vi "PCB Coverage graph.vi"(0 "UpdatedData":T1, 5 "error in (no error)":errorcluster, 6 "XY Graph":refnum<vi>, 7 "index":i32, 9 "Disable Autoscale":bool, 13 "Initialise graph":bool=TRUE) -> (19 "error out":errorcluster)   [LabVIEW 2018, in "Manipulate IPF.lvlib"]
uses:
  Manipulate IPF.lvlib
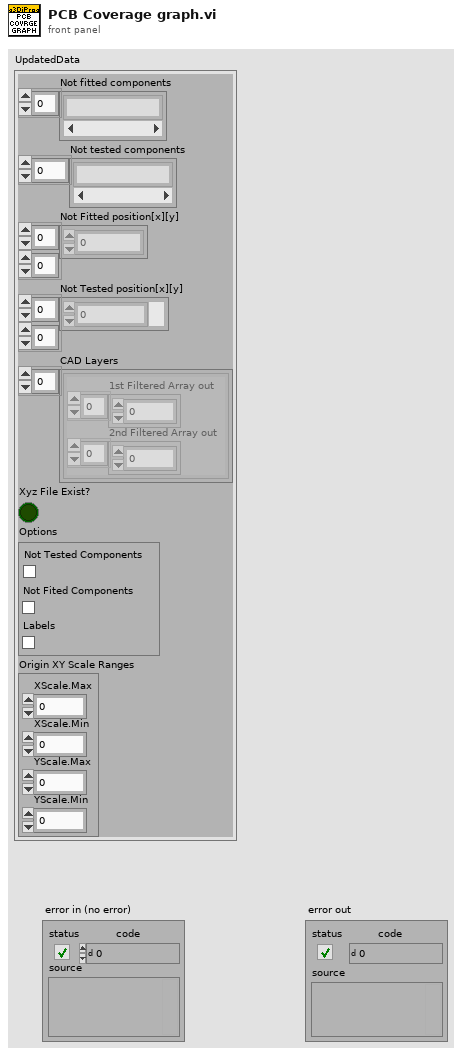
[diagram p1: front panel]
types:
  T1 = cluster{"Not fitted components":string[], "Not tested components":string[], "Not Fitted position[x][y] ":dbl[][], "Not Tested position[x][y]":dbl[][], "CAD Layers":cluster{"1st Filtered Array out":sgl[], "2nd Filtered Array out":sgl[]}[], "Xyz File Exist? ":bool, "Options":cluster{"Enable Not Tested Components":bool, "Enable Not Fited Components":bool, "Enable Labels":bool}, "Origin XY Scale Ranges":cluster{"XScale.Max":dbl, "XScale.Min":dbl, "YScale.Max":dbl, "YScale.Min":dbl}}
  T2 = cluster{"1st Filtered Array out":sgl[], "2nd Filtered Array out":sgl[]}[]
  T3 = cluster{"1st Filtered Array out":sgl[], "2nd Filtered Array out":sgl[]}
  T4 = cluster{"X Array Out":dbl[], "Y Array out":dbl[]}
  T5 = cluster{"X Array Out":dbl[], "Y Array out":dbl[]}[]
  T6 = typedef "LVPoint32TypeDef.ctl" = cluster{"Horizontal":i32, "Vertical":i32}
  T7 = typedef "LVAnnotationListTypeDef.ctl" = cluster{"Name":string, "Color":u32, "Style":u8, "Point Style":u8, "Name Visible":bool, "Allow Drag":bool, "Annotation Mode":u32, "Plot":i32, "Index":i32, "Position":cluster{"X":dbl, "Y":dbl}, "X Scale":u32, "Y Scale":u32, "Show Arrow":bool, "Lock Name":bool, "Plot Area":i32, "Label Offset":cluster{"X":dbl, "Y":dbl}}[]
  T8 = cluster{"Name":string, "Color":u32, "Style":u8, "Point Style":u8, "Name Visible":bool, "Allow Drag":bool, "Annotation Mode":u32, "Plot":i32, "Index":i32, "Position":cluster{"X":dbl, "Y":dbl}, "X Scale":u32, "Y Scale":u32, "Show Arrow":bool, "Lock Name":bool, "Plot Area":i32, "Label Offset":cluster{"X":dbl, "Y":dbl}}
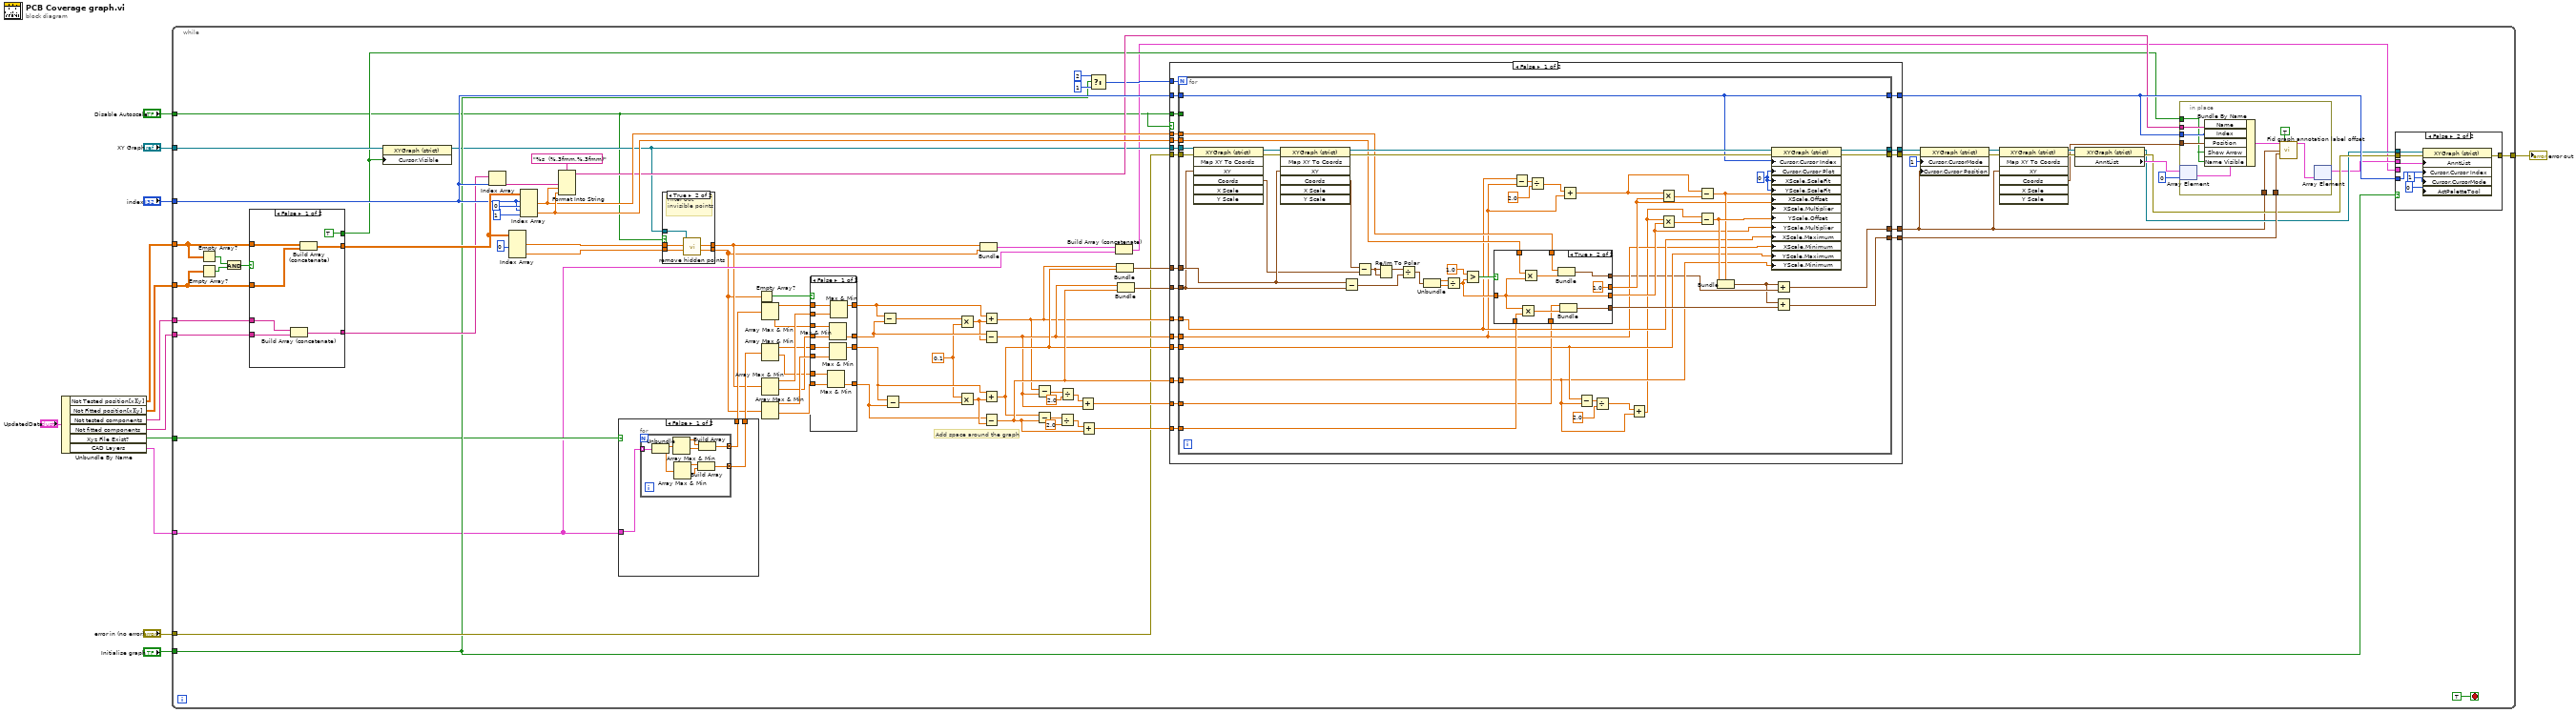
[diagram p0: block diagram]
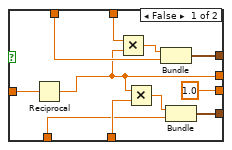
[diagram p2: hidden frame]
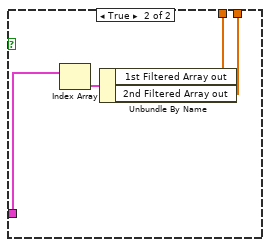
[diagram p4: hidden frame]
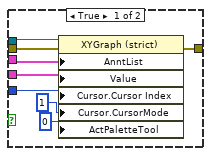
[diagram p7: hidden frame]
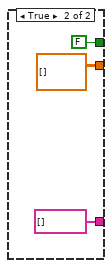
[diagram p8: hidden frame]
diagram:
  n1 = Unbundle By Name("UpdatedData") -> ("Not Tested position[x][y]"=w4:dbl[][], "Not Fitted position[x][y]"=w2:dbl[][], "Not tested components"=w3:string[], "Not fitted components"=w1:string[], "Xyz File Exist?"=w6:bool, "CAD Layers"=w7:T2)
  n2 = while {
    tunnel: "error in (no error)" -> [w71]
    tunnel: w4 -> [w62]
    tunnel: "index" -> [w49]
    tunnel: "XY Graph" -> [w57]
    tunnel: [w64] -> w10
    tunnel: "Initialise graph" -> [w33]
    tunnel: w2 -> [w61]
    tunnel: w3 -> [w54]
    tunnel: w1 -> [w53]
    tunnel: "Disable Autoscale" -> [w14]
    tunnel: w6 -> [w20]
    tunnel: w7 -> [w19]
    stop <- TRUE stop-if-true
    w98 = 0.1
    # "Add space around the graph"
    n3 = Empty Array?(array=w62) -> (empty?=w60:bool)
    n4 = Empty Array?(array=w61) -> (empty?=w59:bool)
    n5 = And(x=w60, y=w59) -> (x .and. y?=w58:bool)
    n6 = case shown="False" w58 {
      tunnel: w62 -> [w264 _]
      tunnel: w61 -> [w263 _]
      tunnel: [w262 dbl[][] []] -> w56
      tunnel: [TRUE FALSE] -> w30
      tunnel: w54 -> [w261 _]
      tunnel: w53 -> [w260 _]
      tunnel: [w259 string[] []] -> w48
      frame False {
        n7 = Build Array (concatenate)(w261, w260) -> (w259:string[])
        n8 = Build Array (concatenate)(w264, w263) -> (w262:dbl[][])
      }
      frame True {
      }
    }
    n9 = property class="XYGraph (strict)"(reference=w57, "Cursor.Visible"=w30) -> (reference out=w24:refnum<vi>)  [unwired: 1 in, 1 out]
    n10 = Index Array(array=w48, index=w49) -> (element=w47:string)
    n11 = Index Array(array=w56, index (col) #1=0 ("index (row)")) -> (element #1=w23:dbl[], element #2=w22:dbl[])  [unwired: 3 in]
    n12 = Index Array(array=w56, index (row) #1=w49, index (col) #1=0 ("index (row)"), index (row) #2=w49, index (col) #2=1 ("index (row)")) -> (element #1=w50:dbl, element #2=w51:dbl)
    n13 = Format Into String(format string="%s  (%.3fmm,%.3fmm)", w47, w50, w51) -> (resulting string=w39:string)  [unwired: 2 in, 1 out]
    n14 = case shown="False" w20 {
      tunnel: [w196 w207] -> w27
      tunnel: [w197 w208] -> w28
      tunnel: w19 -> [w195 w210]
      frame False {
        n15 = for {
          tunnel: w195 -> [w206] mode=indexing
          tunnel: [w202] -> w197 mode=concatenating
          tunnel: [w198] -> w196 mode=concatenating
          n16 = Unbundle(w206) -> ("1st Filtered Array out"=w205:sgl[], "2nd Filtered Array out"=w201:sgl[])
          n17 = Array Max & Min(array=w205) -> (max value=w204:sgl, min value=w203:sgl)  [unwired: 2 out]
          n18 = Array Max & Min(array=w201) -> (max value=w199:sgl, min value=w200:sgl)  [unwired: 2 out]
          n19 = Build Array(w199, w200) -> (w198:sgl[])
          n20 = Build Array(w204, w203) -> (w202:sgl[])
        }
      }
      frame True {
        n21 = Index Array(array=w210) -> (element=w209:T3)  [unwired: 1 in]
        n22 = Unbundle By Name(w209) -> ("1st Filtered Array out"=w208:sgl[], "2nd Filtered Array out"=w207:sgl[])
      }
    }
    n23 = case shown="True" w14 {
      tunnel: w24 -> [_ w217]
      tunnel: w23 -> [w212 w214]
      tunnel: w22 -> [w211 w213]
      tunnel: [w211 w215] -> w15
      tunnel: [w212 w216] -> w16
      frame False {
      }
      frame True {
        # "Filter out invisible points"
        n24 = call "remove hidden points.vi"("Y Array in"=w213, "X Array In"=w214, "XYGraph in"=w217) -> ("Y Array out"=w215:dbl[], "X Array Out"=w216:dbl[])  [unwired: 6 in, 1 out]
      }
    }
    n25 = Empty Array?(array=w15) -> (empty?=w55:bool)
    n26 = Array Max & Min(array=w28) -> (max value=w86:sgl, min value=w87:sgl)  [unwired: 2 out]
    n27 = Array Max & Min(array=w27) -> (max value=w88:sgl, min value=w89:sgl)  [unwired: 2 out]
    n28 = Array Max & Min(array=w16) -> (max value=w90:dbl, min value=w91:dbl)  [unwired: 2 out]
    n29 = Array Max & Min(array=w15) -> (max value=w93:dbl, min value=w92:dbl)  [unwired: 2 out]
    n30 = case shown="False" w55 {
      tunnel: [w229 w230] -> w31
      tunnel: [w228 w231] -> w100
      tunnel: [w227 w232] -> w99
      tunnel: [w226 w233] -> w32
      tunnel: w93 -> [w225 _]
      tunnel: w92 -> [w224 _]
      tunnel: w91 -> [w223 _]
      tunnel: w90 -> [w222 _]
      tunnel: w89 -> [w221 w230]
      tunnel: w88 -> [w220 w231]
      tunnel: w87 -> [w219 w232]
      tunnel: w86 -> [w218 w233]
      frame False {
        n31 = Max & Min(x=w221, y=w224) -> (min(x,y)=w229:dbl)  [unwired: 1 out]
        n32 = Max & Min(x=w219, y=w223) -> (min(x,y)=w227:dbl)  [unwired: 1 out]
        n33 = Max & Min(x=w220, y=w225) -> (max(x,y)=w228:dbl)  [unwired: 1 out]
        n34 = Max & Min(x=w218, y=w222) -> (max(x,y)=w226:dbl)  [unwired: 1 out]
      }
      frame True {
      }
    }
    n35 = Subtract(x=w32, y=w99) -> (x-y=w94:dbl)
    n36 = Subtract(x=w100, y=w31) -> (x-y=w95:dbl)
    n37 = Multiply(x=w94, y=w98) -> (x*y=w96:dbl)
    n38 = Multiply(x=w98, y=w95) -> (x*y=w97:dbl)
    n39 = Bundle("X Array Out"=w16, "Y Array out"=w15) -> (w21:T4)  [unwired: 1 in]
    n40 = Add(x=w32, y=w96) -> (x+y=w74:dbl)
    n41 = Subtract(x=w99, y=w96) -> (x-y=w75:dbl)
    n42 = Add(x=w100, y=w97) -> (x+y=w76:dbl)
    n43 = Subtract(x=w31, y=w97) -> (x-y=w77:dbl)
    n44 = Subtract(x=w74, y=w75) -> (x-y=w80:dbl)
    n45 = Subtract(x=w76, y=w77) -> (x-y=w85:dbl)
    n46 = Divide(x=w85, y=2.0) -> (x/y=w83:dbl)
    n47 = Divide(x=w80, y=2.0) -> (x/y=w82:dbl)
    n48 = Add(x=w82, y=w75) -> (x+y=w78:dbl)
    n49 = Add(x=w83, y=w77) -> (x+y=w79:dbl)
    n50 = Select(t=2, s=w33, f=1) -> (s? t:f=w35:i32)
    n51 = Build Array (concatenate)(w21, w19) -> (w17:T5)
    n52 = Bundle(w74, w76) -> (w72:cluster{dbl, dbl})  [unwired: 1 in]
    n53 = Bundle(w75, w77) -> (w73:cluster{dbl, dbl})  [unwired: 1 in]
    n54 = case shown="False" w14 {
      tunnel: w79 -> [w120 _]
      tunnel: w78 -> [w119 _]
      tunnel: w77 -> [w118 _]
      tunnel: w76 -> [w117 _]
      tunnel: w75 -> [w116 _]
      tunnel: w74 -> [w115 _]
      tunnel: w73 -> [w114 _]
      tunnel: w72 -> [w113 _]
      tunnel: w71 -> [w112 w192]
      tunnel: [w111 w192] -> w66
      tunnel: w51 -> [w110 _]
      tunnel: w50 -> [w109 _]
      tunnel: w49 -> [w108 w194]
      tunnel: [w107 _] -> w42
      tunnel: [w106 w194] -> w41
      tunnel: w35 -> [w105 _]
      tunnel: [w104 w193] -> w26
      tunnel: [w103 _] -> w25
      tunnel: w24 -> [w102 w193]
      tunnel: w14 -> [w101 _]
      frame False {
        n55 = for {
          N: w105 -> [_]
          tunnel: w113 -> [w170]
          tunnel: w114 -> [w169]
          tunnel: w120 -> [w168]
          tunnel: w109 -> [w147]
          tunnel: w110 -> [w148]
          tunnel: w119 -> [w130]
          tunnel: w112 -> [w167]
          tunnel: w102 -> [w166]
          tunnel: [w123] -> w103
          tunnel: [w122] -> w107
          tunnel: [w151] -> w104
          tunnel: [w126] -> w111
          tunnel: w115 -> [w138]
          tunnel: w116 -> [w136]
          tunnel: w117 -> [w129]
          tunnel: w118 -> [w128]
          tunnel: w108 -> [w149]
          tunnel: [w149] -> w106
          tunnel: w101 -> [_]
          w121 = u8 0 ("X Scale.Scale Fit")
          n56 = invoke class="XYGraph (strict)" method="Map XY To Coords"(reference=w166, error in=w167, "XY"=w169) -> (reference out=w165:refnum<vi>, error out=w164:errorcluster, "Coords"=w162:T6)  [unwired: 4 in, 4 out]
          n57 = invoke class="XYGraph (strict)" method="Map XY To Coords"(reference=w165, error in=w164, "XY"=w170) -> (reference out=w152:refnum<vi>, error out=w150:errorcluster, "Coords"=w163:T6)  [unwired: 4 in, 4 out]
          n58 = Subtract(x=w170, y=w169) -> (x-y=w161:cluster{dbl, dbl})
          n59 = Subtract(x=w163, y=w162) -> (x-y=w157:T6)
          n60 = Re/Im To Polar(2:w157, 3:w157) -> (1:w156:cluster{"Horizontal":dbl, "Vertical":dbl})  [unwired: 1 out]
          n61 = Divide(x=w156, y=w161) -> (x/y=w160:cluster{dbl, dbl})
          n62 = Unbundle(w160) -> (w159:dbl, w158:dbl)
          n63 = Divide(x=w159, y=w158) -> (x/y=w153:dbl)
          n64 = Greater?(x=1.0, y=w153) -> (0:w155:bool)
          n65 = case shown="True" w155 {
            tunnel: [w181 w191] -> w125
            tunnel: [w180 w190] -> w143
            tunnel: w168 -> [w173 w188]
            tunnel: w153 -> [w172 w184]
            tunnel: w147 -> [w177 w182]
            tunnel: w148 -> [w178 w185]
            tunnel: [1.0 w184] -> w142
            tunnel: [w171 1.0] -> w141
            tunnel: w130 -> [w174 w186]
            frame False {
              n66 = Reciprocal(x=w172) -> (1/x=w171:dbl)
              n67 = Multiply(x=w177, y=w171) -> (x*y=w176:dbl)
              n68 = Multiply(x=w171, y=w174) -> (x*y=w175:dbl)
              n69 = Bundle(w176, "String"=w178) -> (w181:cluster{dbl, "String":dbl})  [unwired: 1 in]
              n70 = Bundle(w175, w173) -> (w180:cluster{dbl, dbl})  [unwired: 1 in]
            }
            frame True {
              n71 = Multiply(x=w184, y=w188) -> (x*y=w187:dbl)
              n72 = Multiply(x=w185, y=w184) -> (x*y=w183:dbl)
              n73 = Bundle("String"=w182, w183) -> (w191:cluster{"String":dbl, dbl})  [unwired: 1 in]
              n74 = Bundle(w186, w187) -> (w190:cluster{dbl, dbl})  [unwired: 1 in]
            }
          }
          n75 = Subtract(x=w138, y=w136) -> (x-y=w139:dbl)
          n76 = Divide(x=w139, y=2.0) -> (x/y=w137:dbl)
          n77 = Add(x=w137, y=w136) -> (x+y=w135:dbl)
          n78 = Subtract(x=w129, y=w128) -> (x-y=w132:dbl)
          n79 = Divide(x=w132, y=2.0) -> (x/y=w133:dbl)
          n80 = Add(x=w133, y=w128) -> (x+y=w127:dbl)
          n81 = Multiply(x=w135, y=w141) -> (x*y=w134:dbl)
          n82 = Multiply(x=w127, y=w142) -> (x*y=w146:dbl)
          n83 = Subtract(x=w135, y=w134) -> (x-y=w144:dbl)
          n84 = Subtract(x=w127, y=w146) -> (x-y=w145:dbl)
          n85 = Bundle(w144, w145) -> (w124:cluster{dbl, dbl})  [unwired: 1 in]
          n86 = property class="XYGraph (strict)"(reference=w152, error in=w150, "Cursor.Cursor Index"=w149, "Cursor.Cursor Plot"=w121, "XScale.ScaleFit"=w121, "YScale.ScaleFit"=w121, "XScale.Offset"=w144, "XScale.Multiplier"=w141, "YScale.Offset"=w145, "YScale.Multiplier"=w142, "XScale.Maximum"=w138, "XScale.Minimum"=w136, "YScale.Maximum"=w129, "YScale.Minimum"=w128) -> (reference out=w151:refnum<vi>, error out=w126:errorcluster)
          n87 = Add(x=w124, y=w125) -> (x+y=w123:cluster{dbl, dbl})
          n88 = Add(x=w124, y=w143) -> (x+y=w122:cluster{dbl, dbl})
        }
      }
      frame True {
      }
    }
    n89 = property class="XYGraph (strict)"(reference=w26, error in=w66, "Cursor.CursorMode"=u32 1 ("Cursor.Cursor Mode"), "Cursor.Cursor Position"=w25) -> (reference out=w67:refnum<vi>, error out=w68:errorcluster)
    n90 = invoke class="XYGraph (strict)" method="Map XY To Coords"(reference=w67, error in=w68, "XY"=w25) -> (reference out=w46:refnum<vi>, error out=w45:errorcluster, "Coords"=w40:T6)  [unwired: 4 in, 4 out]
    n91 = property class="XYGraph (strict)"(reference=w46, error in=w45) -> (reference out=w37:refnum<vi>, error out=w38:errorcluster, "AnntList"=w44:T7)
    n92 = in-place {
      in-place-border: w40 -> [w242]
      in-place-border: w41 -> [w241]
      in-place-border: w39 -> [w240]
      in-place-border: w42 -> [w237]
      in-place-border: w25 -> [w235]
      in-place-border: w30 -> [w234]
      n93 = in-place-array #1(w44, 0) -> (w243:T8)
      n94 = Bundle By Name(cluster=w243, "Name"=w240, "Index"=w241, "Position"=w242, "Show Arrow"=w234, "Name Visible"=w234) -> (w239:T8)
      n95 = call "Fid graph annotation label offset.vi"("Annotation List"=w239, "Load Graph Centre x, y"=TRUE, "Cursor Position"=w235, "Graph centre"=w237) -> ("Annotation List"=w238:T8)  [unwired: 11 in]
      n96 = in-place-array #1(w238) -> (w29:T7)  [unwired: 1 out]
    }
    n97 = case shown="False" w33 {
      tunnel: w41 -> [w250 w257]
      tunnel: w37 -> [w249 w256]
      tunnel: w38 -> [w248 w255]
      tunnel: w17 -> [w247 _]
      tunnel: [w246 w254] -> w64
      tunnel: w29 -> [w245 w253]
      frame True {
        n98 = property class="XYGraph (strict)"(reference=w249, error in=w248, "AnntList"=w245, "Value"=w247, "Cursor.Cursor Index"=w250, "Cursor.CursorMode"=u32 1 ("Cursor.Cursor Mode"), "ActPaletteTool"=0 ("Palette:Active Tool")) -> (error out=w246:errorcluster)  [unwired: 1 out]
      }
      frame False {
        n99 = property class="XYGraph (strict)"(reference=w256, error in=w255, "AnntList"=w253, "Cursor.Cursor Index"=w257, "Cursor.CursorMode"=u32 1 ("Cursor.Cursor Mode"), "ActPaletteTool"=0 ("Palette:Active Tool")) -> (error out=w254:errorcluster)  [unwired: 1 out]
      }
    }
  }
  "error out" <- w10
